vi "worksheet ignore errors.vi"(8 "error in (no error)":errorcluster, 9 "range":string, 10 "type":u8, 11 "worksheet":u32) -> (0 "error out":errorcluster)   [LabVIEW 2015, in "xlsxwriter.lvlib"]
doc: "void worksheet_ignore_errors(lxw_worksheet worksheet, uint8_t type, const char *range);"
uses:
  xlsxwriter.lvlib
  xlsxwriter.dll
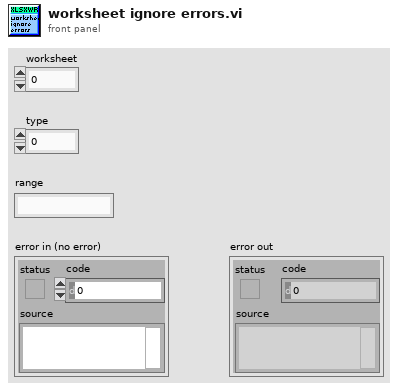
[diagram p1: front panel]
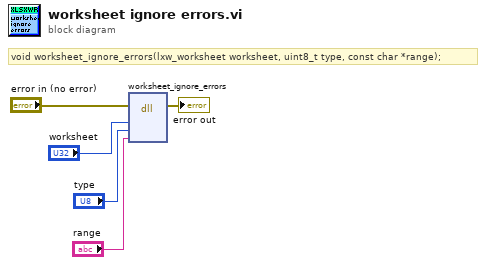
[diagram p0: block diagram]
diagram:
  # "void worksheet_ignore_errors(lxw_worksheet worksheet, uint8_t type, const char *range);"
  n1 = dll-call lib="C:/Users/WDAGUtilityAccount/Desktop/lv_vis_added_cell/xlsxwriter.*" fn="worksheet_ignore_errors"(error in="error in (no error)", "worksheet"="worksheet", "type"="type", "range"="range") -> (error out=→"error out":errorcluster)  [unwired: 6 in, 1 out]
